vi "1553BZhufen-RECV-START.vi"(8 "错误输入（无错误）":errorcluster, 10 "Zhufen":bool, 11 "字节流文件输入":refnum<file>) -> (0 "错误输出":errorcluster)   [LabVIEW 2012]
uses:
  <vilib>/GPower/VIRegister/Library/Convert/ToU8.vi
  <vilib>/GPower/VIRegister/Library/Convert/ToStr.vi
  <vilib>/GPower/VIRegister/Library/Convert/ToU32.vi
  <vilib>/GPower/VIRegister/Library/SubVIs/FindRegisterData.vi
  <vilib>/GPower/VIRegister/Library/SubVIs/ReadSub.vi
  <vilib>/GPower/VIRegister/Library/SubVIs/WriteSub.vi
  <vilib>/GPower/VIRegister/Library/QManager/GetRegisterData.vi
  <vilib>/GPower/Error/Library/SetError.vi
  <vilib>/GPower/Error/Library/FilterCodes.vi
  <vilib>/GPower/Error/Library/Filter/FilterMulti.vi
  <vilib>/GPower/VIRegister/Library/QManager/QManagerAction.vi
  <vilib>/GPower/Error/Library/ErrorType.vi
  <vilib>/GPower/Error/Library/SplitAppended.vi
  <vilib>/GPower/Error/Library/SubVIs/ExplanationToError.vi
  <vilib>/GPower/VIRegister/Library/QManager/GetQName.vi
  <vilib>/GPower/VIRegister/Library/QManager/StartQManager.vi
  <vilib>/Utility/error.llb/Trim Whitespace.vi
  <vilib>/dlg_ctls.llb/Space Constant.vi
  <vilib>/Utility/error.llb/Error Code Database.vi
  <vilib>/GPower/Error/Library/SubVIs/SetStatus.vi
  <vilib>/GPower/Error/Library/AppendErrors.vi
  <vilib>/GPower/Error/Library/Append/AppendSingle.vi
  <vilib>/GPower/VIRegister/VIRegister.lvlib
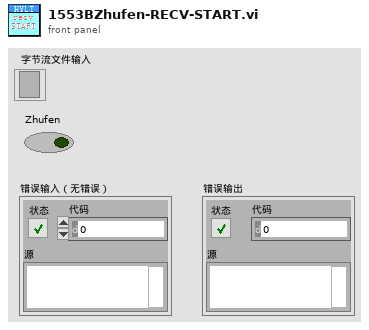
[diagram p1: front panel]
types:
  T1 = cluster{"G1陀螺脉冲数":i32, "G2陀螺脉冲数":i32, "G3陀螺脉冲数":i32, "A1加速度计脉冲数":i16, "A2加速度计脉冲数":i16, "A3加速度计脉冲数":i16, "G1陀螺自检状态":u8, "G1陀螺光路温度":i8, "G2陀螺自检状态":u8, "G2陀螺光路温度":i8, "G3陀螺自检状态":u8, "G3陀螺光路温度":i8, "A1自检状态":u8, "A1幅值":u8, "A2自检状态":u8, "A2幅值":u8, "A3自检状态":u8, "A3幅值":u8, "IF1电路温度":i8, "IF2电路温度":i8, "IF3电路温度":i8, "温控自检字":u8, "加计温度1":i16, "加计温度2":i16, "LTU状态":u8, "帧计数":u8, "G1陀螺光路温度E-2":i16, "G2陀螺光路温度E-2":i16, "G3陀螺光路温度E-2":i16, "G1陀螺电路温度E-2":i16, "G2陀螺电路温度E-2":i16, "G3陀螺电路温度E-2":i16}
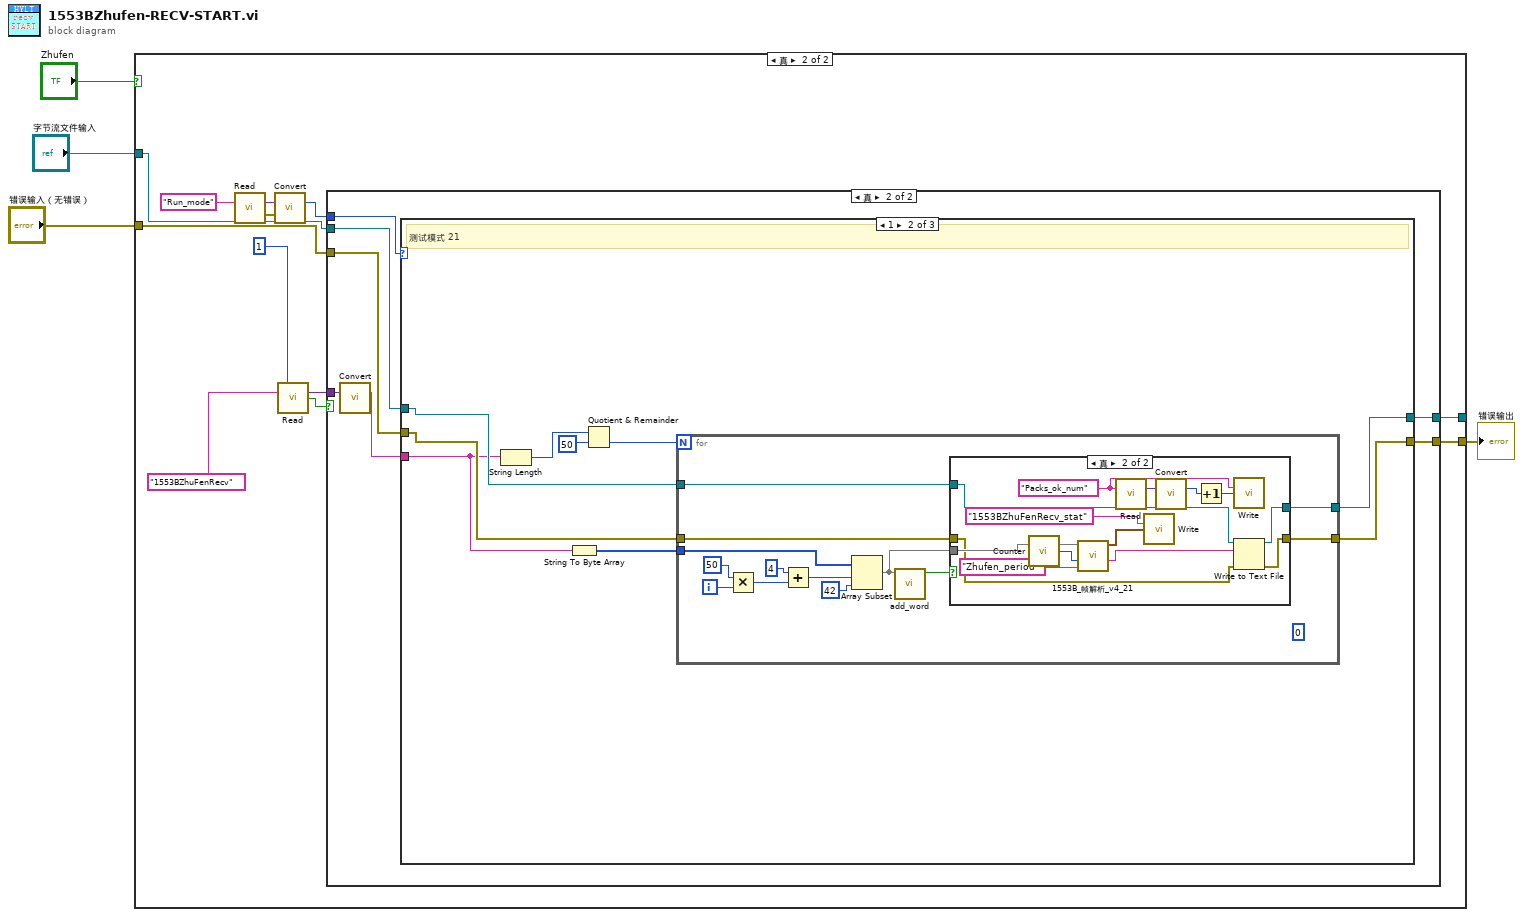
[diagram p0: block diagram]
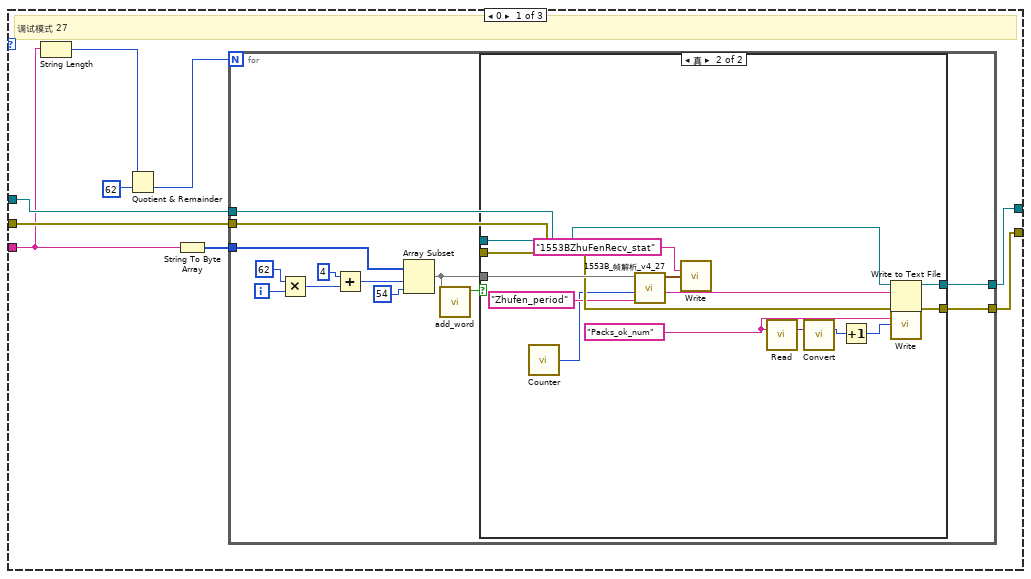
[diagram p4: hidden frame]
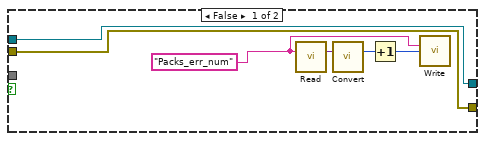
[diagram p5: hidden frame]
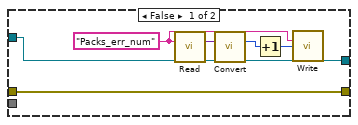
[diagram p6: hidden frame]
diagram:
  n1 = case shown="真" "Zhufen" {
    tunnel: "字节流文件输入" -> [w5 w11]
    tunnel: "错误输入（无错误）" -> [w6 w10]
    tunnel: [w6 w9] -> w4
    tunnel: [w5 w13] -> _
    frame False {
    }
    frame True {
      n2 = call <vilib>:"Read.vi"("Register name"="Run_mode") -> ("Register value"=w14:variant, "Error out"=w8:errorcluster)  [unwired: 11 in, 2 out]
      n3 = call-poly <vilib>:"Convert.vi"("Register value in"=w14, "Error in"=w8) -> ("Register value out"=w12:u8)  [unwired: 12 in, 1 out]
      n4 = call <vilib>:"Read.vi"("Timeout"=1, "Register name"="1553BZhuFenRecv") -> ("Register value"=w17:variant, "Register value read?"=w18:bool)  [unwired: 10 in, 2 out]
      n5 = case shown="真" w18 {
        tunnel: w17 -> [_ w27]
        tunnel: w11 -> [w19 w25]
        tunnel: w12 -> [_ w24]
        tunnel: w10 -> [w20 w23]
        tunnel: [w20 w22] -> w9
        tunnel: [w19 w21] -> w13
        frame False {
        }
        frame True {
          n6 = call-poly <vilib>:"Convert.vi"("Register value in"=w27) -> ("Register value out"=w26:string)  [unwired: 13 in, 1 out]
          n7 = case shown="1" w24 {
            tunnel: w26 -> [w31 w74 _]
            tunnel: w25 -> [w35 w78 w113]
            tunnel: w23 -> [w34 w77 w112]
            tunnel: [w33 w76 w112] -> w22
            tunnel: [w32 w75 w113] -> w21
            frame 0 {
              # "调试模式 27"
              n8 = String Length(string=w31) -> (length=w30:i32)
              n9 = Quotient & Remainder(x=w30, y=62) -> (floor(x/y)=w28:i32)  [unwired: 1 out]
              n10 = String To Byte Array(string=w31) -> (unsigned byte array=w36:u8[])
              n11 = for {
                N: w28 -> [_]
                tunnel: w36 -> [w39]
                tunnel: w35 -> [w48]
                tunnel: w34 -> [w47]
                tunnel: [w46] -> w33
                tunnel: [w45] -> w32
                i -> [w44]
                n12 = Multiply(x=62, y=w44) -> (x*y=w42:i32)
                n13 = Add(x=4 ("索引"), y=w42) -> (x+y=w40:i32)
                n14 = Array Subset(array=w39, index=w40, length=54 ("长度")) -> (w38:u8[])
                n15 = call "add_word.vi"("子数组"=w38) -> ("校验通过"=w37:bool)  [unwired: 10 in]
                n16 = case shown="真" w37 {
                  tunnel: w48 -> [w55 w69]
                  tunnel: w38 -> [_ w68]
                  tunnel: w47 -> [w54 w66]
                  tunnel: [w54 w65] -> w46
                  tunnel: [w55 w64] -> w45
                  frame False {
                    w50 = "Packs_err_num" ("Register name")
                    n17 = call <vilib>:"Read.vi"("Register name"=w50) -> ("Register value"=w53:variant)  [unwired: 11 in, 3 out]
                    n18 = call-poly <vilib>:"Convert.vi"("Register value in"=w53) -> ("Register value out"=w52:u32)  [unwired: 13 in, 1 out]
                    n19 = Increment(x=w52) -> (x+1=w51:u32)
                    n20 = call <vilib>:"Write.vi"("Register name"=w50, "Register value"=w51) -> ()  [unwired: 11 in, 3 out]
                  }
                  frame True {
                    w59 = "Packs_ok_num" ("Register name")
                    n21 = call "Counter.vi"() -> ("Counter"=w56:u64)  [unwired: 1 in]
                    n22 = call "1553B_帧解析_v4_27.vi"("ZhuBeiFen?"="Zhufen_period" ("Register name"), "Counter"=w56, "数组"=w68) -> ("连接的字符串"=w67:string, "输出簇"=w58:T1)  [unwired: 7 in]
                    n23 = call <vilib>:"Write.vi"("Register name"="1553BZhuFenRecv_stat" ("字符串"), "Register value"=w58) -> ()  [unwired: 11 in, 3 out]
                    n24 = call <vilib>:"Read.vi"("Register name"=w59) -> ("Register value"=w63:variant)  [unwired: 11 in, 3 out]
                    n25 = call-poly <vilib>:"Convert.vi"("Register value in"=w63) -> ("Register value out"=w62:u32)  [unwired: 13 in, 1 out]
                    n26 = Increment(x=w62) -> (x+1=w61:u32)
                    n27 = Write to Text File(file (use dialog)=w69, text=w67, error in=w66) -> (refnum out=w64:refnum<file>, error out=w65:errorcluster)  [unwired: 1 in, 1 out]
                    n28 = call <vilib>:"Write.vi"("Register name"=w59, "Register value"=w61) -> ()  [unwired: 11 in, 3 out]
                  }
                }
              }
            }
            frame 1 {
              # "测试模式 21"
              n29 = String Length(string=w74) -> (length=w72:i32)
              n30 = String To Byte Array(string=w74) -> (unsigned byte array=w73:u8[])
              n31 = Quotient & Remainder(x=w72, y=50) -> (floor(x/y)=w70:i32)  [unwired: 1 out]
              n32 = for {
                N: w70 -> [_]
                tunnel: w73 -> [w82]
                tunnel: w78 -> [w90]
                tunnel: w77 -> [w80]
                tunnel: [w89] -> w76
                tunnel: [w88] -> w75
                i -> [w87]
                (unwired) 0 ("索引")
                n33 = Multiply(x=50, y=w87) -> (x*y=w85:i32)
                n34 = Add(x=4 ("索引"), y=w85) -> (x+y=w83:i32)
                n35 = Array Subset(array=w82, index=w83, length=42 ("长度")) -> (w81:u8[])
                n36 = call "add_word.vi"("子数组"=w81) -> ("校验通过"=w79:bool)  [unwired: 10 in]
                n37 = case shown="真" w79 {
                  tunnel: w90 -> [w97 w111]
                  tunnel: [w96 w110] -> w89
                  tunnel: [w97 w109] -> w88
                  tunnel: w81 -> [_ w107]
                  tunnel: w80 -> [w96 w106]
                  frame False {
                    w95 = "Packs_err_num" ("Register name")
                    n38 = call <vilib>:"Read.vi"("Register name"=w95) -> ("Register value"=w94:variant)  [unwired: 11 in, 3 out]
                    n39 = call-poly <vilib>:"Convert.vi"("Register value in"=w94) -> ("Register value out"=w93:u32)  [unwired: 13 in, 1 out]
                    n40 = Increment(x=w93) -> (x+1=w92:u32)
                    n41 = call <vilib>:"Write.vi"("Register name"=w95, "Register value"=w92) -> ()  [unwired: 11 in, 3 out]
                  }
                  frame True {
                    w102 = "Packs_ok_num" ("Register name")
                    n42 = call "Counter.vi"() -> ("Counter"=w98:u64)  [unwired: 1 in]
                    n43 = call "1553B_帧解析_v4_21.vi"("Register name"="Zhufen_period", "Counter"=w98, "数组"=w107) -> ("连接的字符串"=w100:string, "输出簇"=w108:T1)  [unwired: 7 in]
                    n44 = call <vilib>:"Read.vi"("Register name"=w102) -> ("Register value"=w105:variant)  [unwired: 11 in, 3 out]
                    n45 = call <vilib>:"Write.vi"("Register name"="1553BZhuFenRecv_stat" ("字符串"), "Register value"=w108) -> ()  [unwired: 11 in, 3 out]
                    n46 = call-poly <vilib>:"Convert.vi"("Register value in"=w105) -> ("Register value out"=w104:u32)  [unwired: 13 in, 1 out]
                    n47 = Increment(x=w104) -> (x+1=w103:u32)
                    n48 = call <vilib>:"Write.vi"("Register name"=w102, "Register value"=w103) -> ()  [unwired: 11 in, 3 out]
                    n49 = Write to Text File(file (use dialog)=w111, text=w100, error in=w106) -> (refnum out=w109:refnum<file>, error out=w110:errorcluster)  [unwired: 1 in, 1 out]
                  }
                }
              }
            }
            frame 2, Default {
            }
          }
        }
      }
    }
  }
  "错误输出" <- w4
